vi "SIGMOID Vector Elements.vi"(2 "X":T1) -> (16 "sigmoid(X)":T1)   [LabVIEW 2014]
uses:
  <vilib>/Analysis/Matrix/Datatypes/RealMatrix.ctl
  <vilib>/Analysis/Matrix/NI_Matrix.lvlib
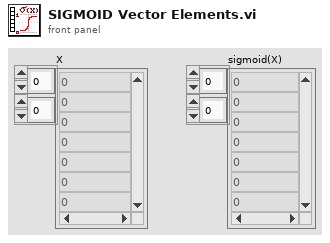
[diagram p1: front panel]
types:
  T1 = typedef "NI_Matrix.lvlib/RealMatrix.ctl" = dbl[][]
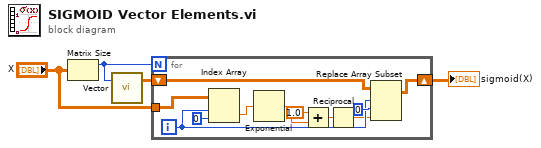
[diagram p0: block diagram]
diagram:
  n1 = Matrix Size(0:"X") -> (1:w3:i32)  [unwired: 1 out]
  n2 = call "Vector.vi"("length"=w3) -> ("Real Matrix (Column Vector)"=w2:T1)  [unwired: 18 in]
  n3 = for {
    N: w3 -> [_]
    tunnel: "X" -> [w12]
    shift-right: [w14] -> w1
    shift-left: w2 -> [w15]
    i -> [w11]
    n4 = Index Array(array=w12, index (row)=w11, index (col)=0) -> (element=w6:dbl)
    n5 = Exponential(1:w6) -> (0:w7:dbl)
    n6 = Add(x=1.0, y=w7) -> (x+y=w9:dbl)
    n7 = Reciprocal(x=w9) -> (1/x=w5:dbl)
    n8 = Replace Array Subset(array=w15, new element=w5, index (row)=w11, index (col)=0 ("disabled index (col)")) -> (w14:T1)
  }
  "sigmoid(X)" <- w1
